vi "LinkNodes.vi"(8 "error in (no error)":errorcluster, 10 "NextNode in":refnum<data-value>, 11 "PreviousNode in":refnum<data-value>) -> (0 "error out":errorcluster, 2 "NextNode out":refnum<data-value>, 3 "PreviousNode out":refnum<data-value>)   [LabVIEW 2014, in "LinkedList.lvlib" / "LinkedList.lvclass"]
doc: "Links two nodes together."
uses:
  <userlib>/AdvancedDataStructures/ClassBased/LinkedList/LinkedList.lvclass
  <userlib>/AdvancedDataStructures/ClassBased/LLNode/LLNode.lvclass
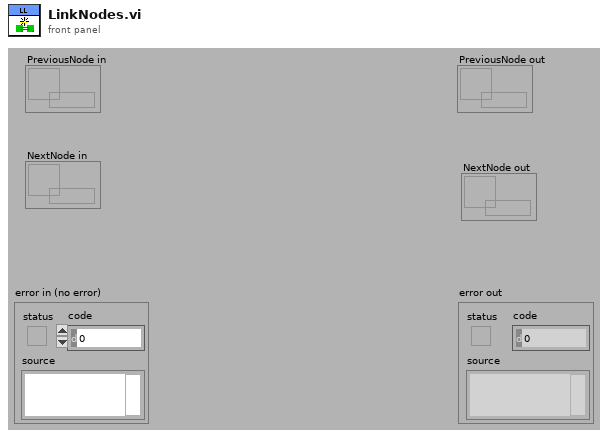
[diagram p1: front panel]
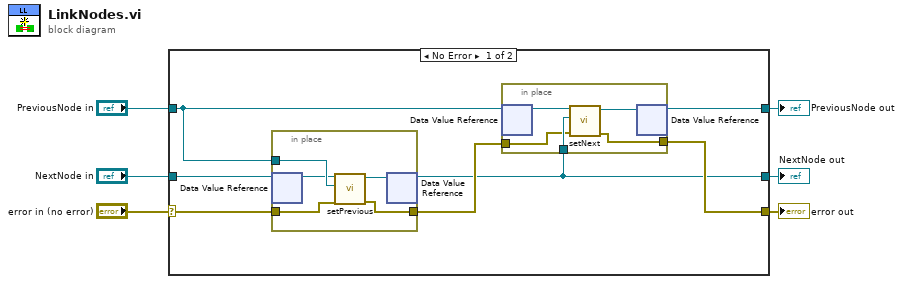
[diagram p0: block diagram]
diagram:
  n1 = case shown="No Error" "error in (no error)" {
    selector: "error in (no error)" -> [w11 w26]
    tunnel: [w9 w26] -> w5
    tunnel: "NextNode in" -> [w13 w24]
    tunnel: "PreviousNode in" -> [w12 w25]
    tunnel: [w8 w25] -> w2
    tunnel: [w7 w24] -> w1
    frame No Error {
      n2 = in-place {
        in-place-border: w12 -> [w22]
        in-place-border: w11 -> [w19]
        in-place-border: [w21] -> w10
        n3 = in-place-dvr #1(w13) -> (w20:refnum<class "LLNode.lvclass">)  [unwired: 1 out]
        n4 = call <userlib>:"setPrevious.vi"("error in (no error)"=w19, "previous"=w22, "LLNode in"=w20) -> ("error out"=w21:errorcluster, "LLNode out"=w23:refnum<class "LLNode.lvclass">)  [unwired: 7 in]
        n5 = in-place-dvr #1(w23) -> (w7:refnum<data-value>)  [unwired: 1 out]
      }
      n6 = in-place {
        in-place-border: w7 -> [w17]
        in-place-border: w10 -> [w14]
        in-place-border: [w16] -> w9
        n7 = in-place-dvr #2(w12) -> (w15:refnum<class "LLNode.lvclass">)  [unwired: 1 out]
        n8 = call <userlib>:"setNext.vi"("error in (no error)"=w14, "next"=w17, "LLNode in"=w15) -> ("error out"=w16:errorcluster, "LLNode out"=w18:refnum<class "LLNode.lvclass">)  [unwired: 7 in]
        n9 = in-place-dvr #2(w18) -> (w8:refnum<data-value>)  [unwired: 1 out]
      }
    }
    frame Error {
    }
  }
  "error out" <- w5
  "PreviousNode out" <- w2
  "NextNode out" <- w1
